vi "NI VeriStand - Add Output Underflow Count Channel.vi"(5 "Highlight? (F)":bool, 8 "error in (no error)":errorcluster, 10 "Channel Name":string, 11 "Parent Ref in":T1 format="%.0x") -> (0 "error out":errorcluster, 1 "Channel Ref":T1 format="%.0x", 3 "Parent Ref out":T1 format="%.0x")   [LabVIEW 2020, in "Custom Device Offline API.lvlib"]
uses:
  <vilib>/NI VeriStand/Custom Device Offline API/Custom Device Offline API.lvlib
  <vilib>/NI VeriStand/Custom Device API/Custom Device Item Ref.ctl
  NationalInstruments.VeriStand.SystemDefinitionAPI
  <vilib>/NI VeriStand/Custom Device API/Custom Device API.lvlib
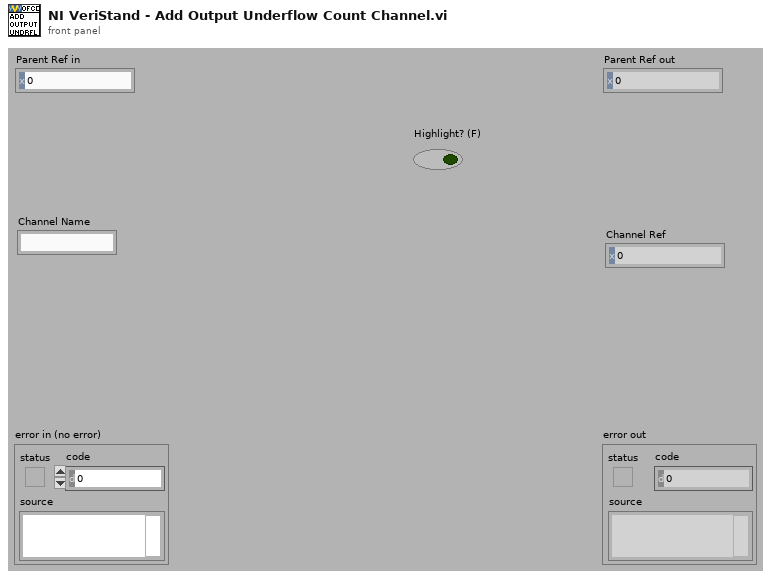
[diagram p1: front panel]
types:
  T1 = typedef "Custom Device API.lvlib/Custom Device Item Ref.ctl" = u64
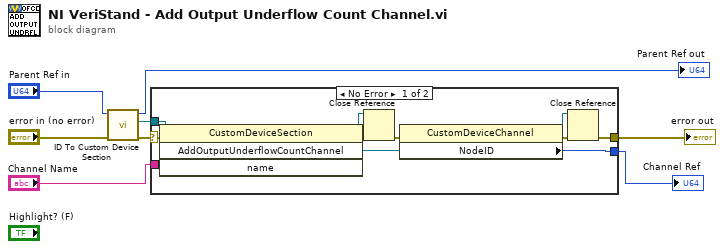
[diagram p0: block diagram]
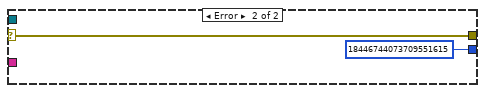
[diagram p2: hidden frame]
diagram:
  n1 = call <vilib>:"ID To Custom Device Section.vi"("error in (no error)"="error in (no error)", "ID in"="Parent Ref in") -> ("error out"=w6:errorcluster, "Section"=w5:refnum<k24>, "ID out"=→"Parent Ref out":u64)  [unwired: 7 in]
  n2 = case shown="No Error" w6 {
    selector: w6 -> [w18 w21]
    tunnel: w5 -> [w19 _]
    tunnel: "Channel Name" -> [w17 _]
    tunnel: [w12 T1 18446744073709551615 ("Section Ptr")] -> w3
    tunnel: [w9 w21] -> w2
    frame No Error {
      n3 = invoke class="CustomDeviceSection" method="AddOutputUnderflowCountChannel"(reference=w19, error in=w18, "name"=w17) -> (reference out=w15:refnum<k24>, error out=w16:errorcluster, "AddOutputUnderflowCountChannel"=w14:refnum<k24>)  [unwired: 1 in, 1 out]
      n4 = Close Reference(reference=w15, error in (no error)=w16) -> (error out=w13:errorcluster)
      n5 = property class="CustomDeviceChannel"(reference=w14, error in=w13) -> (reference out=w10:refnum<k24>, error out=w11:errorcluster, "NodeID"=w12:u64)
      n6 = Close Reference(reference=w10, error in (no error)=w11) -> (error out=w9:errorcluster)
    }
    frame Error {
    }
  }
  "error out" <- w2
  "Channel Ref" <- w3
